vi "Data Min-Max.vi"(0 "VISA resource name":refnum<visa-resource-name>, 7 "Input (0: A)":u16(ring) items=["A", "B", "C", "D"], 11 "error in (no error)":errorcluster) -> (4 "VISA resource name out":refnum<visa-resource-name>, 8 "Min Value":dbl min=-1500.0 max=300000.0 step=0.0001 format="%^.4e", 10 "Max Value":dbl min=-1500.0 max=300000.0 step=0.0001 format="%^.4e", 15 "error out":errorcluster)   [LabVIEW 2019, in "Lake Shore Cryotronics 340.lvlib"]
doc: "This VI querys the instrument for an inputs min/max readings."
uses:
  Lake Shore Cryotronics 340.lvlib
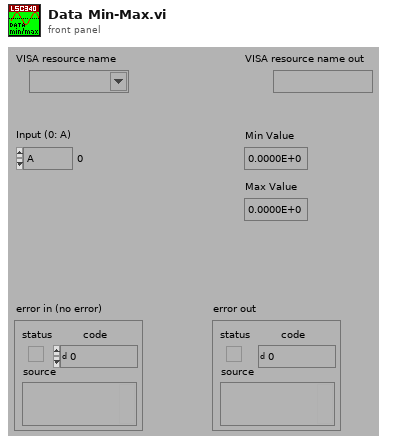
[diagram p1: front panel]
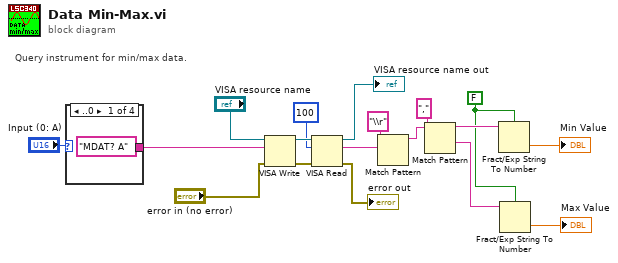
[diagram p0: block diagram]
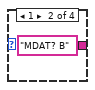
[diagram p2: hidden frame]
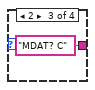
[diagram p3: hidden frame]
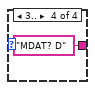
[diagram p4: hidden frame]
diagram:
  w1 = FALSE ("use system decimal point (T)")
  # "Query instrument for min/max data."
  n1 = case shown="..0" "Input (0: A)" {
    tunnel: ["MDAT? A" "MDAT? B" "MDAT? C" "MDAT? D"] -> w2
    frame ..0 {
    }
    frame 1 {
    }
    frame 2 {
    }
    frame 3.. {
    }
  }
  n2 = VISA Write(VISA resource name="VISA resource name", write buffer=w2, error in (no error)="error in (no error)") -> (VISA resource name out=w15:refnum<visa-resource-name>, error out=w14:errorcluster)  [unwired: 1 out]
  n3 = VISA Read(VISA resource name=w15, byte count=100, error in (no error)=w14) -> (VISA resource name out=→"VISA resource name out":refnum<visa-resource-name>, read buffer=w12:string, error out=→"error out":errorcluster)  [unwired: 1 out]
  n4 = Match Pattern(string=w12, regular expression="\\r") -> (before substring=w9:string)  [unwired: 1 in, 3 out]
  n5 = Match Pattern(string=w9, regular expression=",") -> (before substring=w8:string, after substring=w7:string)  [unwired: 1 in, 2 out]
  n6 = Fract/Exp String To Number(use system decimal point (T)=w1, string=w8) -> (number=→"Min Value":dbl)  [unwired: 2 in, 1 out]
  n7 = Fract/Exp String To Number(use system decimal point (T)=w1, string=w7) -> (number=→"Max Value":dbl)  [unwired: 2 in, 1 out]
